vi "Background Loop Step.vi"(8 "error in (no error)":errorcluster, 10 "Action":T1, 11 "Lockin Digitizer in":refnum<class "Lockin Digitizer.lvclass">) -> (0 "error out":errorcluster, 1 "Next step delay":i32, 2 "Action out":T1=enum."Stop", 3 "Lockin Digitizer out":refnum<class "Lockin Digitizer.lvclass">, 4 "Result":refnum<class "Acquired Result.lvclass">)   [LabVIEW 2021, in "Lockin Digitizer.lvclass"]
uses:
  Lockin Digitizer.lvclass
  Lockin Digitizer.lvclass/Lockin Digitizer.ctl
  Pulse Recorder/Pulse Recorder.lvclass
  NHMFL_Core/Libraries/Instruments/Pulse Driver/Lockin Digitizer Driver/Lockin Digitizer Driver.lvclass
  Worker/Background Loop Action.ctl
  NHMFL_Core/Libraries/Instruments/Results/Acquired Result/Acquired Result.lvclass
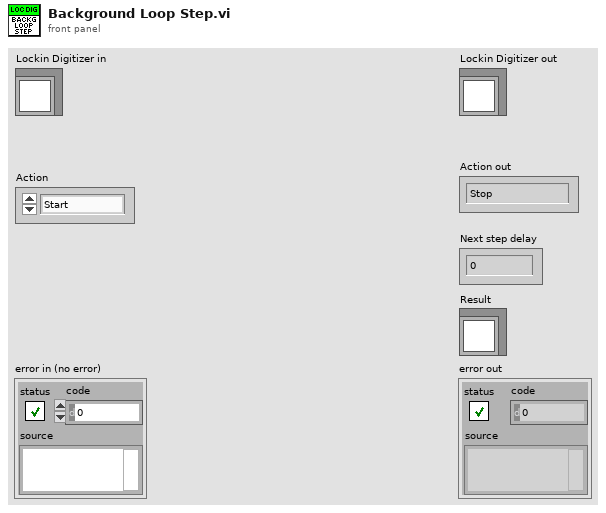
[diagram p1: front panel]
types:
  T1 = typedef "Background Loop Action.ctl" = enum16{"Start", "Continue", "Stop"}
  T2 = typedef "Lockin Digitizer Configuration.ctl" = cluster{"Post-trigger delay":dbl, "Post-trigger duration":dbl, "Rate":dbl, "Ranges":dbl[], "Re-name channels":string[], "Active channels":string, "External\nclock":bool, "Frequencies":dbl[], "Time\nconstant":dbl, "Output \namplitudes":dbl[], "Input\nchannles":string[]}
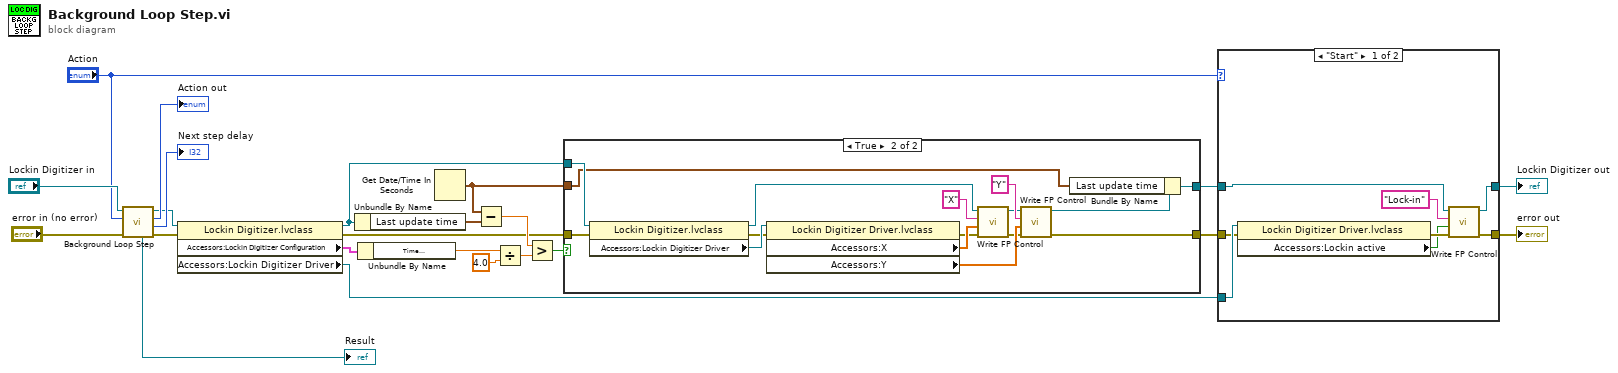
[diagram p0: block diagram]
diagram:
  n1 = call-parent "Background Loop Step.vi"("error in (no error)"="error in (no error)", "Action"="Action", "Instrument Actor in"="Lockin Digitizer in") -> ("error out"=w23:errorcluster, "Next step delay"=→"Next step delay":i32, "Action out"=→"Action out":T1, "Instrument Actor out"=w18:refnum<class "Lockin Digitizer.lvclass">, "Result"=→"Result":refnum<class "Acquired Result.lvclass">)  [unwired: 4 in]
  n2 = property class="Lockin Digitizer.lvclass"(reference=w18, error in=w23) -> (reference out=w10:refnum<class "Lockin Digitizer.lvclass">, error out=w7:errorcluster, "Accessors:Lockin Digitizer Configuration"=w17:T2, "Accessors:Lockin Digitizer Driver"=w8:refnum<class "Lockin Digitizer Driver.lvclass">)
  n3 = Unbundle By Name(w10) -> ("Last update time"=w14:timestamp)
  n4 = Unbundle By Name(w17) -> ("Time\nconstant"=w16:dbl)
  n5 = Get Date/Time In Seconds() -> (seconds since 1Jan1904=w9:timestamp)
  n6 = Subtract(x=w9, y=w14) -> (x-y=w13:dbl)
  n7 = Divide(x=w16, y=4.0) -> (x/y=w12:dbl)
  n8 = Greater?(x=w13, y=w12) -> (0:w11:bool)
  n9 = case shown="True" w11 {
    tunnel: w10 -> [w25 w41]
    tunnel: w7 -> [w24 w40]
    tunnel: w9 -> [_ w30]
    tunnel: [w25 w29] -> w5
    tunnel: [w24 w28] -> w4
    frame False {
    }
    frame True {
      n10 = property class="Lockin Digitizer.lvclass"(reference=w41, error in=w40) -> (reference out=w39:refnum<class "Lockin Digitizer.lvclass">, error out=w26:errorcluster, "Accessors:Lockin Digitizer Driver"=w27:refnum<class "Lockin Digitizer Driver.lvclass">)
      n11 = property class="Lockin Digitizer Driver.lvclass"(reference=w27, error in=w26) -> (error out=w32:errorcluster, "Accessors:X"=w36:dbl[], "Accessors:Y"=w35:dbl[])  [unwired: 1 out]
      n12 = call-dynamic "Write FP Control.vi"("error in (no error)"=w32, "Control Value"=w36, "Control Name"="X", "Measure Object in"=w39) -> ("error out"=w34:errorcluster, "Measure Object out"=w33:refnum<class "Lockin Digitizer.lvclass">)  [unwired: 6 in]
      n13 = call-dynamic "Write FP Control.vi"("error in (no error)"=w34, "Control Value"=w35, "Control Name"="Y", "Measure Object in"=w33) -> ("error out"=w28:errorcluster, "Measure Object out"=w31:refnum<class "Lockin Digitizer.lvclass">)  [unwired: 6 in]
      n14 = Bundle By Name(cluster=w31, "Last update time"=w30) -> (w29:refnum<class "Lockin Digitizer.lvclass">)
    }
  }
  n15 = case shown="\"Start\"" "Action" {
    tunnel: w8 -> [w49 _]
    tunnel: w4 -> [w48 w51]
    tunnel: w5 -> [w43 w50]
    tunnel: [w44 w51] -> w3
    tunnel: [w42 w50] -> w2
    frame "Start" {
      n16 = property class="Lockin Digitizer Driver.lvclass"(reference=w49, error in=w48) -> (error out=w47:errorcluster, "Accessors:Lockin active"=w45:bool)  [unwired: 1 out]
      n17 = call-dynamic "Write FP Control.vi"("error in (no error)"=w47, "Control Value"=w45, "Control Name"="Lock-in", "Measure Object in"=w43) -> ("error out"=w44:errorcluster, "Measure Object out"=w42:refnum<class "Lockin Digitizer.lvclass">)  [unwired: 6 in]
    }
    frame "Continue", Default {
    }
  }
  "error out" <- w3
  "Lockin Digitizer out" <- w2
